vi "Test Skipped Passes.vi"(11 "Test Case In":refnum<class "API Pass Output.lvclass">) -> (0 "error out":errorcluster, 3 "Test Case Out":refnum<class "API Pass Output.lvclass">)   [LabVIEW 2020, in "API Pass Output.lvclass"]
uses:
  API Pass Output.lvclass
  C:/Program Files (x86)/National Instruments/LabVIEW 2020/vi.lib/Astemes/LUnit/Test Case.lvclass
  <vilib>/Astemes/LUnit/Test Case.lvclass/Test Case.ctl
  <vilib>/Astemes/LUnit/Core/LUnit Test Case/Private/Append Fail Result.vi
  <vilib>/Astemes/LUnit/Core/LUnit Test Case/Private/Append Pass Result.vi
  <vilib>/Astemes/LUnit/Core/LUnit Test Case/Private/Run In UI.vi
  <vilib>/Utility/error.llb/Clear Errors.vi
  source/Framework/Execution API/Execution API.lvclass
  <vilib>/Astemes/LUnit/Test Case.lvclass
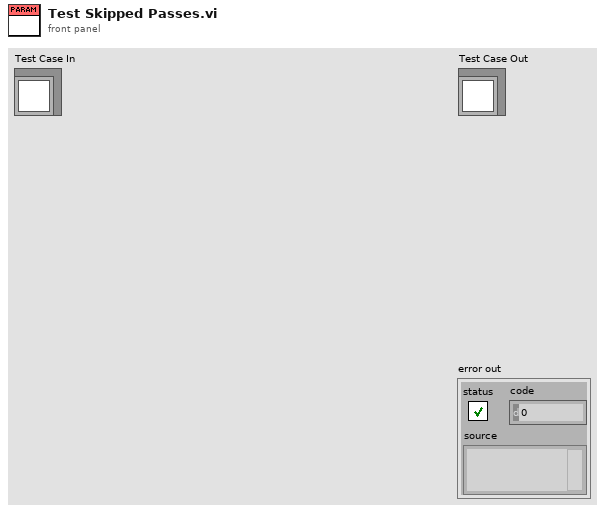
[diagram p1: front panel]
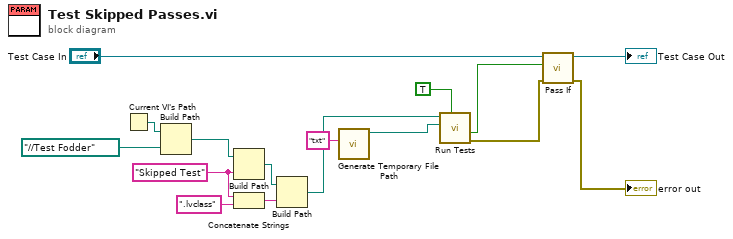
[diagram p0: block diagram]
diagram:
  w2 = "Skipped Test"
  n1 = Current VI's Path() -> (path=w10:path)
  n2 = Build Path(base path=w10, name or relative path=path "../../Test Fodder") -> (appended path=w8:path)
  n3 = Build Path(base path=w8, name or relative path=w2) -> (appended path=w6:path)
  n4 = Concatenate Strings(w2, ".lvclass" ("string")) -> (w5:string)
  n5 = Build Path(base path=w6, name or relative path=w5) -> (appended path=w4:path)
  n6 = call <vilib>:"Generate Temporary File Path.vi"("Temporary File Extension (tmp)"="txt") -> ("Unique Temporary File Path"=w13:path)  [unwired: 9 in, 1 out]
  n7 = call "Run Tests.vi"("Run Tests In Parallel? (T)"=TRUE, "Report Output path"=w13, "Project, Library, or Test Class Path"=w4) -> ("error out"=w12:errorcluster, "All Passed?"=w3:bool)  [unwired: 6 in, 1 out]
  n8 = call <vilib>:"Pass If.vi"("error in (no error)"=w12, "Pass?"=w3, "LUnit Test Case In"="Test Case In") -> ("error out"=→"error out":errorcluster, "LUnit Test Case Out"=→"Test Case Out":refnum<class "API Pass Output.lvclass">)  [unwired: 7 in]
